vi "例程22-二进制文件的写入.vi"() -> ()   [LabVIEW 2016]
uses:
  <vilib>/Analysis/NI_AALBase.lvlib
panel:
  out "写入文件数据":dbl[](graph)
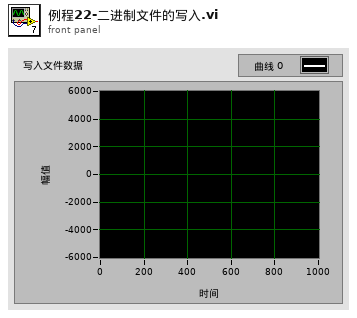
[diagram p1: front panel]
types:
  T1 = enum16{"big-endian, network order", "native, host order", "little-endian"}
  T2 = enum16{"open", "replace", "create", "open or create", "replace or create", "replace or create with confirmation"}
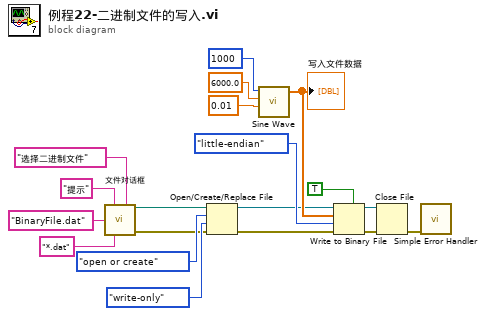
[diagram p0: block diagram]
diagram:
  n1 = call "文件对话框"("prompt"="提示", "button label"="选择二进制文件", "default name"="BinaryFile.dat", "pattern (all files)"="*.dat") -> ("selected path"=w18:path, "error out"=w5:errorcluster)  [unwired: 8 in, 2 out]
  n2 = Open/Create/Replace File(file path (use dialog)=w18, error in=w5, operation (0:open)=T2."open or create" ("操作(0:open)"), access (0:read/write)=enum16{"read/write", "read-only", "write-only"}."write-only" ("权限(0:read/write)")) -> (refnum out=w1:refnum<file>, error out=w2:errorcluster)  [unwired: 2 in, 1 out]
  n3 = call <vilib>:"Sine Wave.vi"("samples"=1000, "amplitude"=6000.0, "frequency"=0.01 ("amplitude")) -> ("sine wave"=w6:dbl[])  [unwired: 2 in, 2 out]
  "写入文件数据" <- w6
  n4 = Write to Binary File(file (use dialog)=w1, data=w6, error in=w2, 5:TRUE ("预置数组或字符串大小？ (T)"), 9:T1."little-endian" ("字节顺序(0:big-endian, network order)")) -> (refnum out=w8:refnum<file>, error out=w9:errorcluster)  [unwired: 1 in, 1 out]
  n5 = Close File(refnum=w8, error in=w9) -> (error out=w7:errorcluster)  [unwired: 1 out]
  n6 = call <vilib>:"Simple Error Handler.vi"("error in (no error)"=w7) -> ()  [unwired: 4 in, 5 out]
